vi "dOD calculation.vi"(7 "Test":T1={"Config"={"Amplification Factor"=2.0, "100% Reflectance Standard"=2.0, "Calculation Method"=enum."Reflectance", "Option to discard new data?"=FALSE, "Mode"=enum."Spectrum", "Number of Averages"=0, "B Test?"=FALSE}, "Indicators"={"DAQ Background Level (V)"=2.0, "A-Test Counter"=2, "B-Test Counter"=2, "Type"=enum."A-Test", "Scope Background Level (Amps)"=2.0, "TAS only?"=FALSE}} {"Config"."Number of Averages" min=0}, 8 "error in":errorcluster, 9 "Waveform Name":string, 10 "Debug Waveform Read In":dbl[][](array[numeric]), 11 "waveform":waveform(dbl)) -> (0 "error out":errorcluster, 2 "Debug Waveform Read Out":dbl[][](array[numeric]), 3 "dOD waveform":waveform(dbl))   [LabVIEW 2017, in "Processing.lvlib"]
uses:
  Processing.lvlib
  System Control/CTLs/Test params.ctl
  System Control/CTLs/Test Controls.ctl
  System Control/CTLs/Test indicators.ctl
  System Control/CTLs/Test Type.ctl
  System Control/Main controller.lvlib
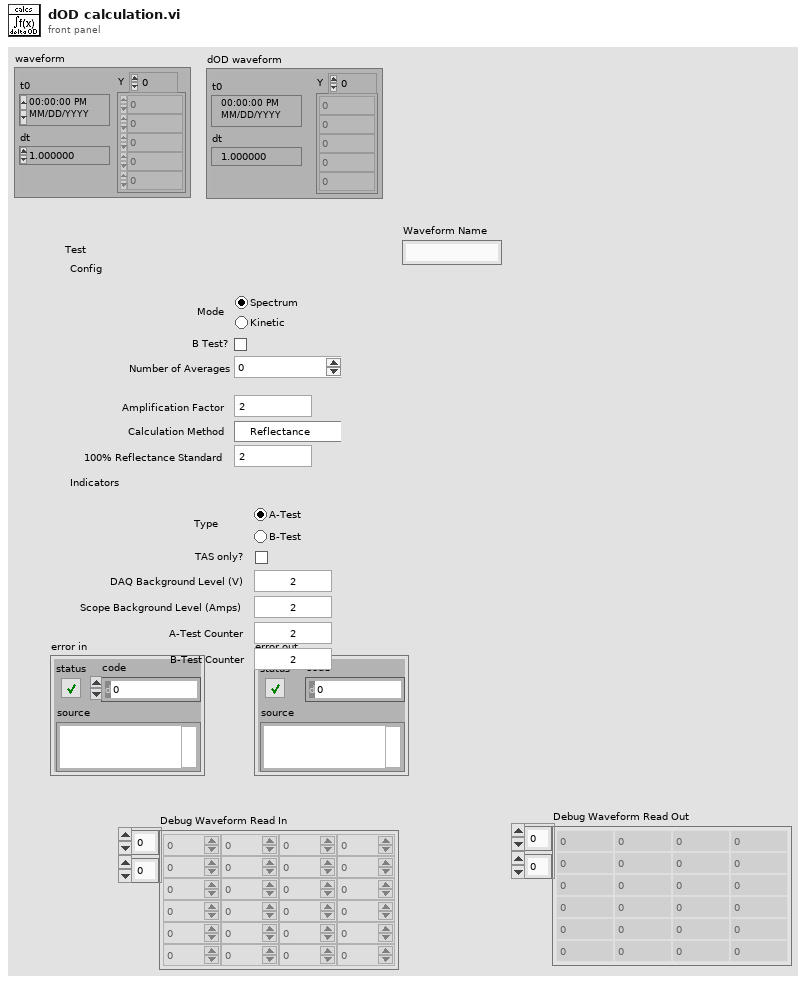
[diagram p1: front panel]
types:
  T1 = typedef "Main controller.lvlib/Test params.ctl" = cluster{"Config":T2, "Indicators":T3}
  T2 = typedef "Main controller.lvlib/Test Controls.ctl" = cluster{"Amplification Factor":dbl, "100% Reflectance Standard":dbl, "Calculation Method":enum16{"Reflectance", "Transmission", "Kubelka-Munk"}, "Option to discard new data?":bool, "Mode":enum32{"Spectrum", "Kinetic"}, "Number of Averages":i32, "B Test?":bool}
  T3 = typedef "Main controller.lvlib/Test indicators.ctl" = cluster{"DAQ Background Level (V)":dbl, "A-Test Counter":i32, "B-Test Counter":i32, "Type":T4, "Scope Background Level (Amps)":dbl, "TAS only?":bool}
  T4 = typedef "Main controller.lvlib/Test Type.ctl" = enum32{"A-Test", "B-Test"}
  T5 = enum16{"Reflectance", "Transmission", "Kubelka-Munk"}
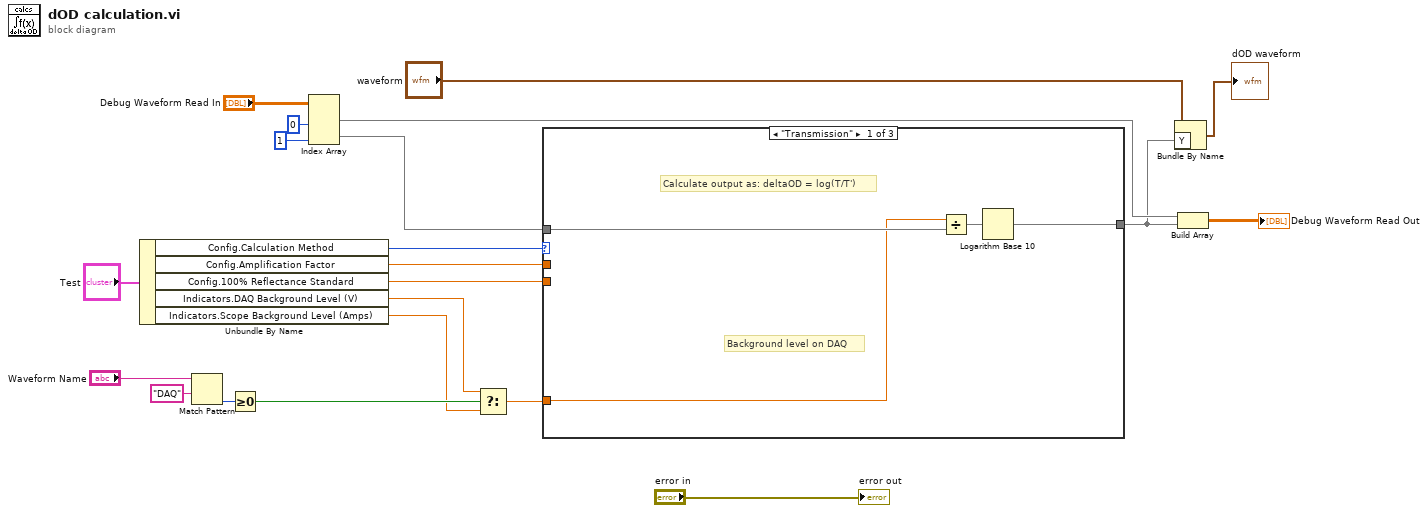
[diagram p0: block diagram]
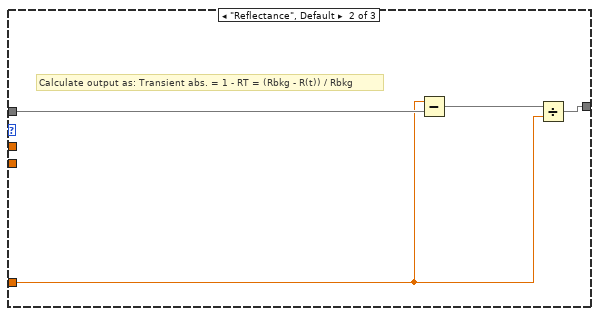
[diagram p2: hidden frame]
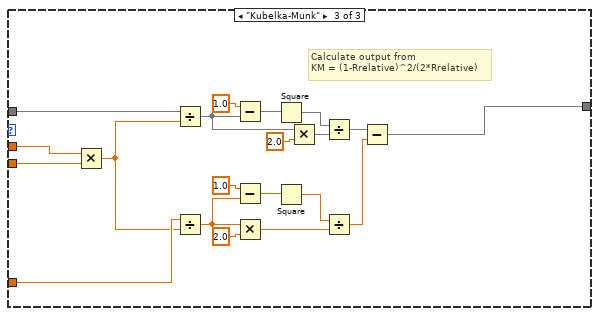
[diagram p3: hidden frame]
diagram:
  n1 = Unbundle By Name("Test") -> ("Config.Calculation Method"=w18:T5, "Config.Amplification Factor"=w9:dbl, "Config.100% Reflectance Standard"=w19:dbl, "Indicators.DAQ Background Level (V)"=w2:dbl, "Indicators.Scope Background Level (Amps)"=w1:dbl)
  n2 = Match Pattern(string="Waveform Name", regular expression="DAQ") -> (offset past match=w6:i32)  [unwired: 1 in, 3 out]
  n3 = Greater Or Equal To 0?(x=w6) -> (x >= 0?=w4:bool)
  n4 = Index Array(array="Debug Waveform Read In", index (col) #1=0 ("disabled index (col)"), index (col) #2=1 ("index (col)")) -> (element #1=w14:dbl[], element #2=w3:dbl[])  [unwired: 2 in]
  n5 = Select(t=w2, s=w4, f=w1) -> (s? t:f=w5:dbl)
  n6 = case shown="\"Transmission\"" w18 {
    tunnel: w3 -> [w24 w29 w49]
    tunnel: [w23 w27 w42] -> w10
    tunnel: w5 -> [w22 w26 w33]
    tunnel: w9 -> [_ _ w32]
    tunnel: w19 -> [_ _ w31]
    frame "Transmission" {
      # "Background level on DAQ"
      # "Calculate output as: deltaOD = log(T/T')"
      n7 = Divide(x=w22, y=w24) -> (x/y=w25:dbl[])
      n8 = Logarithm Base 10(1:w25) -> (0:w23:dbl[])
    }
    frame "Reflectance", Default {
      # "Calculate output as: Transient abs. = 1 - RT = (Rbkg - R(t)) / Rbkg"
      n9 = Subtract(x=w26, y=w29) -> (x-y=w28:dbl[])
      n10 = Divide(x=w28, y=w26) -> (x/y=w27:dbl[])
    }
    frame "Kubelka-Munk" {
      # "Calculate output from\nKM = (1-Rrelative)^2/(2*Rrelative)"
      n11 = Multiply(x=w32, y=w31) -> (x*y=w30:dbl)
      n12 = Divide(x=w49, y=w30) -> (x/y=w35:dbl[])
      n13 = Divide(x=w33, y=w30) -> (x/y=w44:dbl)
      n14 = Subtract(x=1.0, y=w35) -> (x-y=w37:dbl[])
      n15 = Subtract(x=1.0, y=w44) -> (x-y=w47:dbl)
      n16 = Multiply(x=w44, y=2.0) -> (x*y=w45:dbl)
      n17 = Square(x=w37) -> (x^2=w38:dbl[])
      n18 = Square(x=w47) -> (x^2=w46:dbl)
      n19 = Multiply(x=w35, y=2.0) -> (x*y=w39:dbl[])
      n20 = Divide(x=w38, y=w39) -> (x/y=w34:dbl[])
      n21 = Divide(x=w46, y=w45) -> (x/y=w41:dbl)
      n22 = Subtract(x=w34, y=w41) -> (x-y=w42:dbl[])
    }
  }
  n23 = Bundle By Name(cluster="waveform", "Y"=w10) -> (→"dOD waveform":waveform(dbl))
  n24 = Build Array(w14, w10) -> (→"Debug Waveform Read Out":dbl[][])
  "error out" <- "error in"
